vi "Find Missing Elements in Array (Double).vi"(10 "Full Array":dbl[](array[numeric]), 11 "Partial Array":dbl[](array[numeric])) -> (3 "Missing Elements":dbl[](array[numeric]))   [LabVIEW 2016]
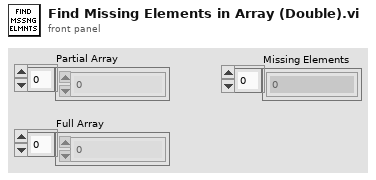
[diagram p1: front panel]
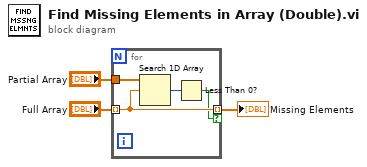
[diagram p0: block diagram]
diagram:
  n1 = for {
    tunnel: "Full Array" -> [w5] mode=indexing
    tunnel: "Partial Array" -> [w7]
    tunnel: [w5] -> w3 mode=indexing if=w4
    n2 = Search 1D Array(1D array=w7, element=w5) -> (index of element=w6:i32)  [unwired: 1 in]
    n3 = Less Than 0?(x=w6) -> (x < 0?=w4:bool)
  }
  "Missing Elements" <- w3
